vi "Azimut_Solar.vi"(1 "Hora Solar":dbl, 2 "Angulo Horario":dbl, 3 "Declinacion":dbl, 4 "n":dbl, 5 "Segundos":i32, 6 "Minutos":i32, 7 "Grados":i32) -> (0 "Azimut Solar":dbl)   [LabVIEW 2020]
panel:
  out "Pre Azimut":dbl
  # "Latitud"
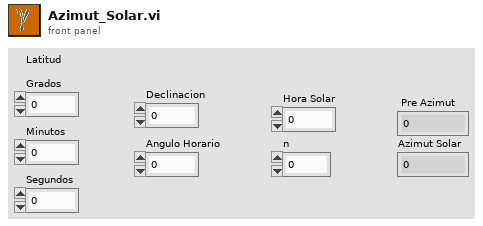
[diagram p1: front panel]
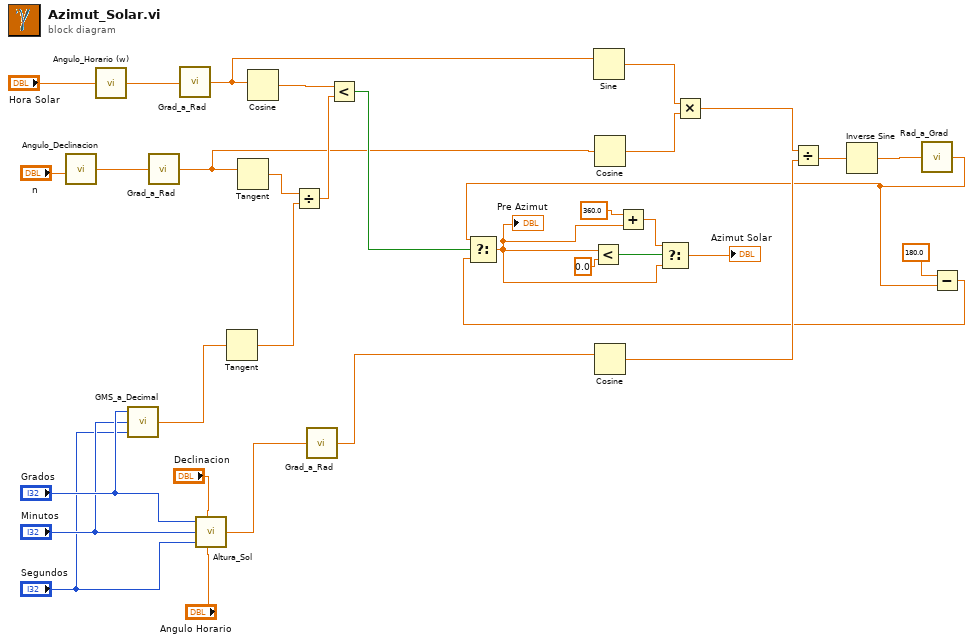
[diagram p0: block diagram]
diagram:
  n1 = call "Angulo_Declinacion.vi"("n"="n") -> ("Declinación"=w11:dbl)
  n2 = call "Angulo_Horario (w).vi"("Hora Solar"="Hora Solar") -> ("Ángulo Horario (w)"=w13:dbl)
  n3 = call "GMS_a_Decimal.vi"("Segundos"="Segundos", "Minutos"="Minutos", "Grados"="Grados") -> ("Decimal"=w2:dbl)
  n4 = call "Grad_a_Rad.vi"("Grados"=w11) -> ("Radianes"=w10:dbl)
  n5 = call "Grad_a_Rad.vi"("Grados"=w13) -> ("Radianes"=w12:dbl)
  n6 = call "Altura_Sol.vi"("Grados"="Grados", "Declinación"="Declinacion", "Minutos"="Minutos", "Segundos"="Segundos", "Ángulo Horario"="Angulo Horario") -> ("Altura del Sol"=w9:dbl)
  n7 = Tangent(1:w2) -> (0:w1:dbl)
  n8 = Tangent(1:w10) -> (0:w31:dbl)
  n9 = Cosine(x=w12) -> (cos(x)=w34:dbl)
  n10 = Divide(x=w31, y=w1) -> (x/y=w30:dbl)
  n11 = call "Grad_a_Rad.vi"("Grados"=w9) -> ("Radianes"=w8:dbl)
  n12 = Less?(x=w34, y=w30) -> (x < y?=w29:bool)
  n13 = Sine(x=w12) -> (sin(x)=w26:dbl)
  n14 = Cosine(x=w10) -> (cos(x)=w25:dbl)
  n15 = Cosine(x=w8) -> (cos(x)=w23:dbl)
  n16 = Multiply(x=w26, y=w25) -> (x*y=w24:dbl)
  n17 = Divide(x=w24, y=w23) -> (x/y=w22:dbl)
  n18 = Inverse Sine(1:w22) -> (0:w7:dbl)
  n19 = call "Rad_a_Grad.vi"("Radianes"=w7) -> ("Grados"=w6:dbl)
  n20 = Subtract(x=180.0, y=w6) -> (x-y=w20:dbl)
  n21 = Select(t=w6, s=w29, f=w20) -> (s? t:f=w16:dbl)
  "Pre Azimut" <- w16
  n22 = Less?(x=w16, y=0.0) -> (x < y?=w18:bool)
  n23 = Add(x=360.0, y=w16) -> (x+y=w15:dbl)
  n24 = Select(t=w15, s=w18, f=w16) -> (s? t:f=→"Azimut Solar":dbl)
